vi "Write Paired Module UID.vi"(8 "error in (no error)":errorcluster, 10 "Paired Module UID":string, 11 "E2E Tag Exchange configuration in":refnum<class "E2E Tag Exchange configuration.lvclass">) -> (0 "error out":errorcluster, 3 "E2E Tag Exchange configuration out":refnum<class "E2E Tag Exchange configuration.lvclass">)   [LabVIEW 2015, in "E2E Tag Exchange configuration.lvclass"]
uses:
  E2E Tag Exchange configuration.lvclass
  E2E Tag Exchange configuration.lvclass/E2E Tag Exchange configuration.ctl
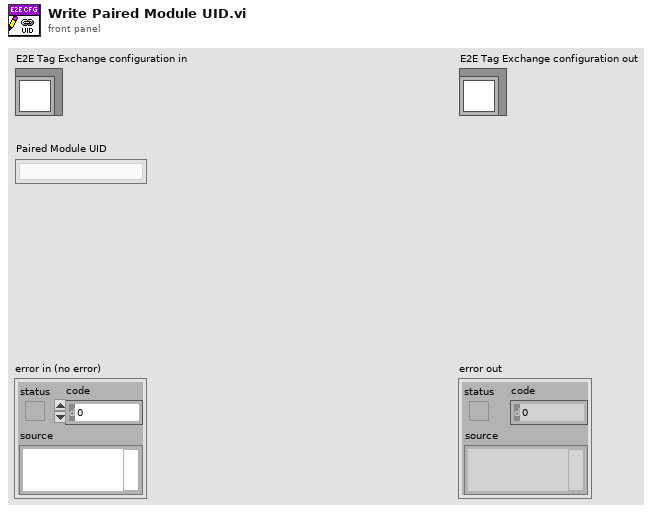
[diagram p1: front panel]
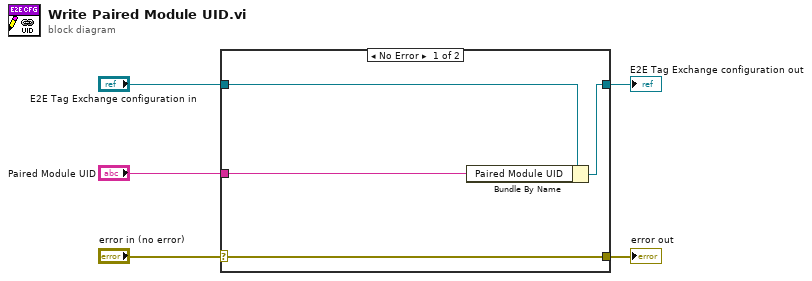
[diagram p0: block diagram]
diagram:
  n1 = case shown="No Error" "error in (no error)" {
    selector: "error in (no error)" -> [w9 w10]
    tunnel: [w9 w10] -> w4
    tunnel: [w7 w11] -> w2
    tunnel: "E2E Tag Exchange configuration in" -> [w8 w11]
    tunnel: "Paired Module UID" -> [w6 _]
    frame No Error {
      n2 = Bundle By Name(cluster=w8, "Paired Module UID"=w6) -> (w7:refnum<class "E2E Tag Exchange configuration.lvclass">)
    }
    frame Error {
    }
  }
  "error out" <- w4
  "E2E Tag Exchange configuration out" <- w2
